vi "LKIF_DataStorageGetData.vi"(8 "error in (no error)":errorcluster {"code" format="%x"}, 10 "NumOutBuffer":i32=1, 11 "OutNo (0: OUT1)":i32) -> (0 "error out":errorcluster {"code" format="%x"}, 2 "NumReceived":i32, 3 "OutBuffer":T1[](array[typedef]) {"LKIF_FLOATRESULT" items=["VALID", "RANGEOVER_P", "RANGEOVER_N", "WAITING"]})   [LabVIEW 2024, in "Keyence LK-G3000.lvlib"]
uses:
  Keyence LK-G3000.lvlib
  clusters/LKIF_FLOATVALUE.ctl
  enums/LKIF_FLOATRESULT.ctl
  Keyance Demo Code/Keyence LK-G3000/LkIF.dll
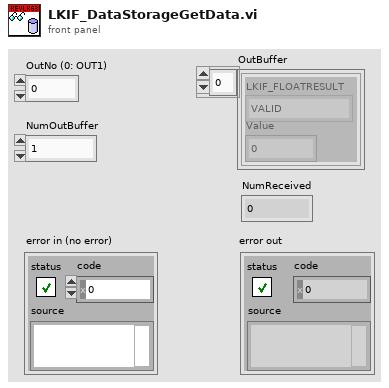
[diagram p1: front panel]
types:
  T1 = typedef "Keyence LK-G3000.lvlib/LKIF_FLOATVALUE.ctl" = cluster{"LKIF_FLOATRESULT":T2, "Value":sgl}
  T2 = typedef "Keyence LK-G3000.lvlib/LKIF_FLOATRESULT.ctl" = i32
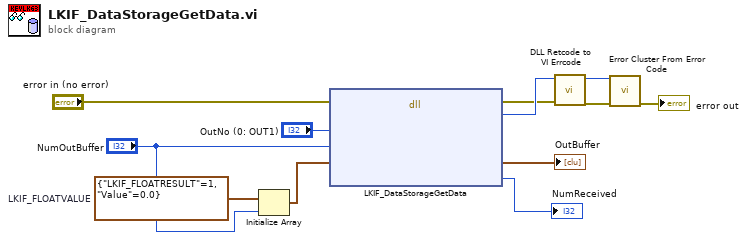
[diagram p0: block diagram]
diagram:
  w8 = T1 {"LKIF_FLOATRESULT"=1, "Value"=0.0}  # LKIF_FLOATVALUE
  n1 = Initialize Array(w8, "NumOutBuffer") -> (w7:T1[])
  n2 = dll-call lib="C:/Users/ff107/OneDrive/Documents/GitHub/PWC-OLS/Hardware Interface/Keyance Demo Code/Keyence LK-G3000/LkIF.dll" fn="LKIF_DataStorageGetData"(error in="error in (no error)", "OutNo"="OutNo (0: OUT1)", "NumOutBuffer"="NumOutBuffer", "OutBuffer"=w7) -> (error out=w2:errorcluster, "RC"=w3:i32, "OutBuffer"=→"OutBuffer":T1[], "NumReceived"=→"NumReceived":i32)  [unwired: 5 in, 1 out]
  n3 = call "DLL Retcode to VI Errcode.vi"("error in (no error)"=w2, "DLL Retcode"=w3) -> ("error out"=w12:errorcluster, "VI Errcode"=w11:i32)  [unwired: 8 in]
  n4 = call <vilib>:"Error Cluster From Error Code.vi"("error in (no error)"=w12, "error code (0)"=w11) -> ("error out"=→"error out":errorcluster)  [unwired: 7 in]
